vi "Get FRU Cluster.vi"(6 "Write Delay Between Pages (ms)":u32, 7 "FRU Type":T3, 8 "error in (no error)":errorcluster, 10 "Unique FRU Input":T1, 11 "CSV Path":path) -> (0 "error out":errorcluster, 2 "FRU Cluster":T2={"Address Byte"=0, "Number of Bytes"=0, "Page Size in Bytes"=128, "Data Byte"=[], "Write Delay Between Pages (ms)"=4} {"Data Byte" format="%02x"; "Address Byte" format="%04x"})   [LabVIEW 2016]
doc: "Get the FRU write array and its content (address byte and data byte) from CSV"
uses:
  Type Definitions/FRU Type.ctl
  Type Definitions/I2C Data Cluster.ctl
  Type Definitions/Unique FRU Input.ctl
  <vilib>/Utility/file.llb/Read Delimited Spreadsheet (string).vi
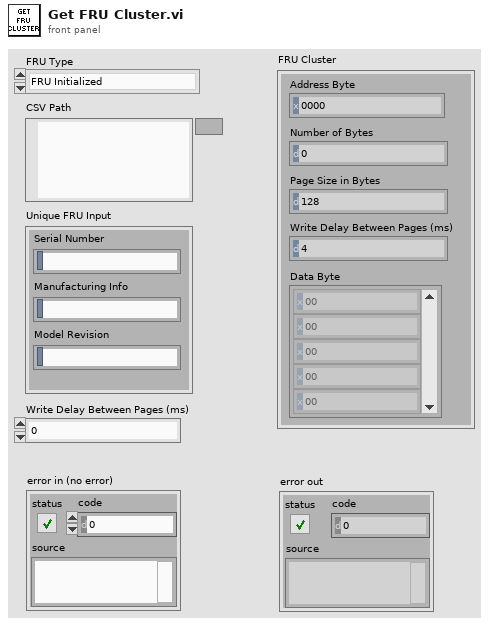
[diagram p1: front panel]
types:
  T1 = typedef "Unique FRU Input.ctl" = cluster{"Serial Number":string, "Manufacturing Info":string, "Model Revision":string}
  T2 = typedef "I2C Data Cluster.ctl" = cluster{"Address Byte":u16, "Number of Bytes":u32, "Page Size in Bytes":u32, "Data Byte":u8[], "Write Delay Between Pages (ms)":u32}
  T3 = typedef "FRU Type.ctl" = enum16{"FRU Initialized", "EEROM Write Protect", "EEPROM Version", "ADI Data Set (Ph-2 GUI)", "Manufacturer's Name", "Product Name", "Serial Number", "Manufacturing Info", "Model Revision", "Alarm Enable", "SCM Internal Temp Limit", "SCM Average Percentage Temp Limit", "PSU1 Iout Limit", "PSU1 Internal Temp Limit", "PSU1 Vin High Limit", "PSU1 Vin Low Limit", "PSU1 Average Percentage Iout Limit", "PSU2 Iout Limit", "PSU2 Internal Temp Limit", "PSU2 Vin High Limit", "PSU2 Vin Low Limit", "PSU2 Average Percentage Iout Limit", "EEPROM Unmodified"}
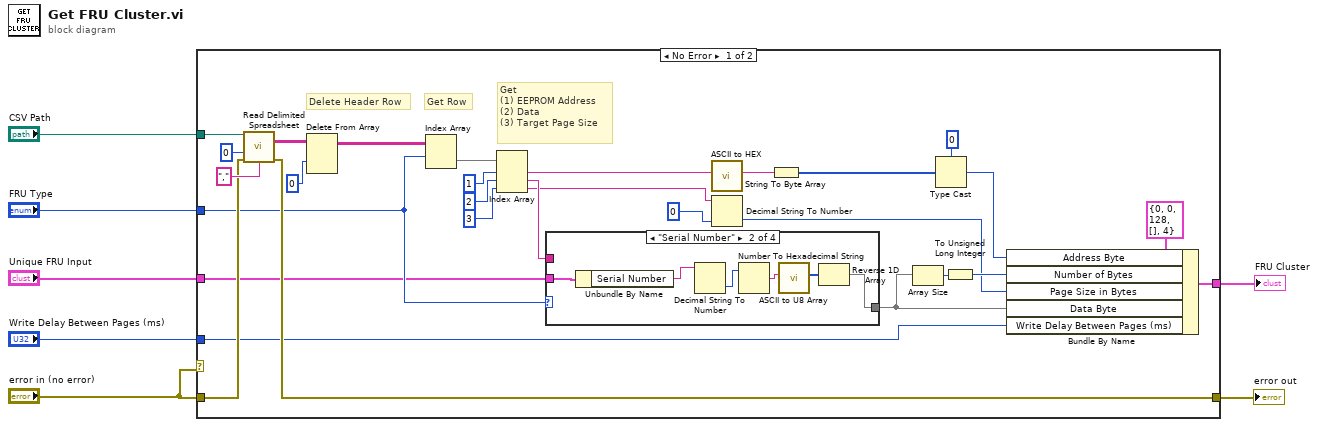
[diagram p0: block diagram]
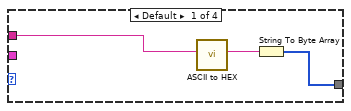
[diagram p2: hidden frame]
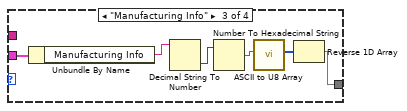
[diagram p3: hidden frame]
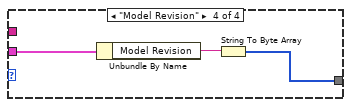
[diagram p4: hidden frame]
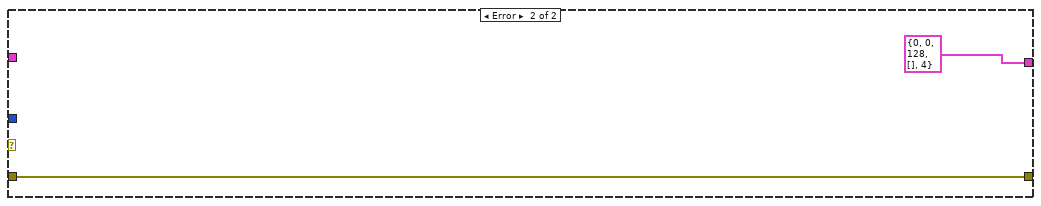
[diagram p5: hidden frame]
diagram:
  n1 = case shown="No Error" "error in (no error)" {
    tunnel: "FRU Type" -> [w23 _]
    tunnel: "CSV Path" -> [w34 _]
    tunnel: "error in (no error)" -> [w32 w56]
    tunnel: [w33 w56] -> w5
    tunnel: "Unique FRU Input" -> [w18 _]
    tunnel: [w14 T2 {"Address Byte"=0, "Number of Bytes"=0, "Page Size in Bytes"=128, "Data Byte"=[], "Write Delay Between Pages (ms)"=4} ("FRU Cluster")] -> w3
    tunnel: "Write Delay Between Pages (ms)" -> [w8 _]
    frame No Error {
      # "Get \n(1) EEPROM Address \n(2) Data \n(3) Target Page Size"
      # "Delete Header Row"
      # "Get Row"
      n2 = call-poly <vilib>:"Read Delimited Spreadsheet.vi"("file path (dialog if empty)"=w34, "start of read offset (chars.:0)"=0, "error in (no error)"=w32, "delimiter (\\t)"="," ("delimiter (\\t)")) -> ("all rows"=w31:string[][], "error out"=w33:errorcluster)  [unwired: 6 in, 4 out]
      n3 = Delete From Array(array=w31, index (row)=0) -> (array with subset deleted=w29:string[][])  [unwired: 2 in, 1 out]
      n4 = Index Array(array=w29, index (row)=w23) -> (element=w24:string[])  [unwired: 1 in]
      n5 = Index Array(array=w24, index #1=1 ("index"), index #2=2 ("index"), index #3=3 ("index")) -> (element #1=w26:string, element #2=w25:string, element #3=w11:string)
      n6 = case shown="\"Serial Number\"" w23 {
        tunnel: [w38 w42 w48 w54] -> w12
        tunnel: w25 -> [w37 _ _ _]
        tunnel: w18 -> [_ w41 w47 w53]
        frame Default {
          n7 = call "ASCII to HEX.vi"("ASCII String"=w37) -> ("Hex String"=w39:string)  [unwired: 10 in]
          n8 = String To Byte Array(string=w39) -> (unsigned byte array=w38:u8[])
        }
        frame "Serial Number" {
          n9 = Unbundle By Name(w41) -> ("Serial Number"=w40:string)
          n10 = Decimal String To Number(string=w40) -> (number=w45:i32)  [unwired: 2 in, 1 out]
          n11 = Number To Hexadecimal String(2:w45) -> (0:w44:string)  [unwired: 1 in]
          n12 = call "ASCII to U8 Array.vi"("ASCII String"=w44) -> ("U8 Array"=w43:u8[])  [unwired: 10 in]
          n13 = Reverse 1D Array(array=w43) -> (reversed array=w42:u8[])
        }
        frame "Manufacturing Info" {
          n14 = Unbundle By Name(w47) -> ("Manufacturing Info"=w46:string)
          n15 = Decimal String To Number(string=w46) -> (number=w51:i32)  [unwired: 2 in, 1 out]
          n16 = Number To Hexadecimal String(2:w51) -> (0:w50:string)  [unwired: 1 in]
          n17 = call "ASCII to U8 Array.vi"("ASCII String"=w50) -> ("U8 Array"=w49:u8[])  [unwired: 10 in]
          n18 = Reverse 1D Array(array=w49) -> (reversed array=w48:u8[])
        }
        frame "Model Revision" {
          n19 = Unbundle By Name(w53) -> ("Model Revision"=w52:string)
          n20 = String To Byte Array(string=w52) -> (unsigned byte array=w54:u8[])
        }
      }
      n21 = call "ASCII to HEX.vi"("ASCII String"=w26) -> ("Hex String"=w21:string)  [unwired: 10 in]
      n22 = Decimal String To Number(string=w11, default (0L)=u32 0 ("Page Size in Bytes")) -> (number=w9:u32)  [unwired: 1 in, 1 out]
      n23 = String To Byte Array(string=w21) -> (unsigned byte array=w20:u8[])
      n24 = Array Size(array=w12) -> (size(s)=w22:i32)
      n25 = Type Cast(type=u16 0 ("number"), x=w20) -> (*(type *) &x=w15:u16)
      n26 = To Unsigned Long Integer(number=w22) -> (unsigned 32bit integer=w16:u32)
      n27 = Bundle By Name(cluster=T2 {"Address Byte"=0, "Number of Bytes"=0, "Page Size in Bytes"=128, "Data Byte"=[], "Write Delay Between Pages (ms)"=4} ("FRU Cluster"), "Address Byte"=w15, "Number of Bytes"=w16, "Page Size in Bytes"=w9, "Data Byte"=w12, "Write Delay Between Pages (ms)"=w8) -> (w14:T2)
    }
    frame Error {
    }
  }
  "error out" <- w5
  "FRU Cluster" <- w3
